vi "uTTA_Send.vi"(7 "Send String":string, 8 "error in (no error)":errorcluster, 10 "TX Termination(\\n)":string="\n", 11 "VISA Refnum in":refnum<visa-resource-name>) -> (0 "error out":errorcluster, 3 "VISA Refnum out":refnum<visa-resource-name>)   [LabVIEW 2021]
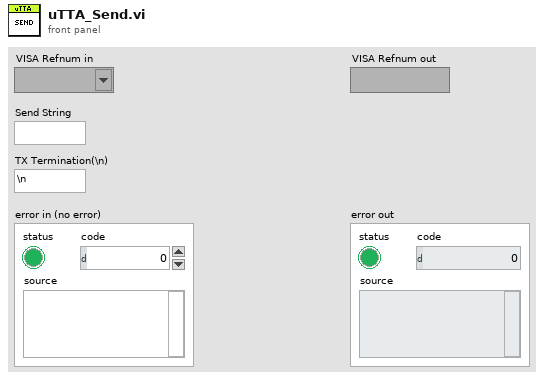
[diagram p1: front panel]
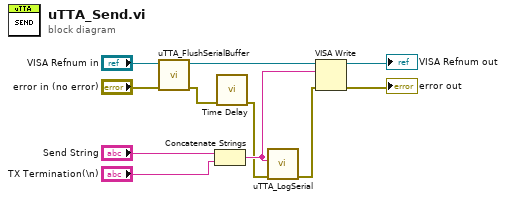
[diagram p0: block diagram]
diagram:
  n1 = call "uTTA_FlushSerialBuffer.vi"("error in (no error)"="error in (no error)", "VISA Refnum in"="VISA Refnum in") -> ("error out"=w5:errorcluster, "VISA Refnum out"=w6:refnum<visa-resource-name>)  [unwired: 4 in]
  n2 = Concatenate Strings("Send String", "TX Termination(\\n)") -> (w9:string)
  n3 = call "Time Delay"("error in (no error)"=w5) -> ("error out"=w2:errorcluster)  [unwired: 10 in]
  n4 = call "uTTA_LogSerial.vi"("error in"=w2, "Data_Sent"=w9) -> ("error out"=w1:errorcluster)  [unwired: 5 in]
  n5 = VISA Write(VISA resource name=w6, write buffer=w9, error in (no error)=w1) -> (VISA resource name out=→"VISA Refnum out":refnum<visa-resource-name>, error out=→"error out":errorcluster)  [unwired: 1 out]
